vi "Control.vi"(8 "DAQ Status":T1, 11 "UI Refs":T6) -> (0 "WaveGen Action":T5, 1 "WaveGen Params":T4, 4 "DAQ Params":T2, 6 "DAQ Action":T3)   [LabVIEW 2020, in "DAQ AO SFP.lvlib"]
uses:
  DAQ AO SFP.lvlib
  UI Refs.ctl
  <extravilib>/ChannelInstances/Flex-t'WaveGen.lvlib-Gen Action.ctl'/))Channel.ctl
  WaveGen/Gen Action.ctl
  <extravilib>/ChannelInstances/Flex-t'WaveGen.lvlib-Gen Params.ctl'/))Channel.ctl
  WaveGen/Gen Params.ctl
  WaveGen/Timing Params.ctl
  WaveGen/Signal Params.ctl
  WaveGen/Shape.ctl
  <extravilib>/ChannelInstances/Flex-t'DAQmx AO.lvlib-Action.ctl'/))Channel.ctl
  DAQmx AO/Action.ctl
  <extravilib>/ChannelInstances/Flex-t'DAQmx AO.lvlib-Params.ctl'/))Channel.ctl
  DAQmx AO/Params.ctl
  <extravilib>/ChannelInstances/Flex-t'DAQmx AO.lvlib-Status.ctl'/))Channel.ctl
  DAQmx AO/Status.ctl
  <extravilib>/ChannelInstances/Flex-t'DAQmx AO.lvlib-Status.ctl'/Event Data.ctl
  <extravilib>/ChannelInstances/Flex-t'DAQmx AO.lvlib-Status.ctl'.lvlib
  DAQmx AO/DAQmx AO.lvlib
  WaveGen/WaveGen.lvlib
  <extravilib>/ChannelInstances/Flex-t'DAQmx AO.lvlib-Params.ctl'.lvlib
  <extravilib>/ChannelInstances/Flex-t'WaveGen.lvlib-Gen Params.ctl'.lvlib
  <extravilib>/ChannelInstances/Flex-t'DAQmx AO.lvlib-Action.ctl'.lvlib
  <extravilib>/ChannelInstances/Flex-t'WaveGen.lvlib-Gen Action.ctl'.lvlib
panel:
  out "Valid":bool
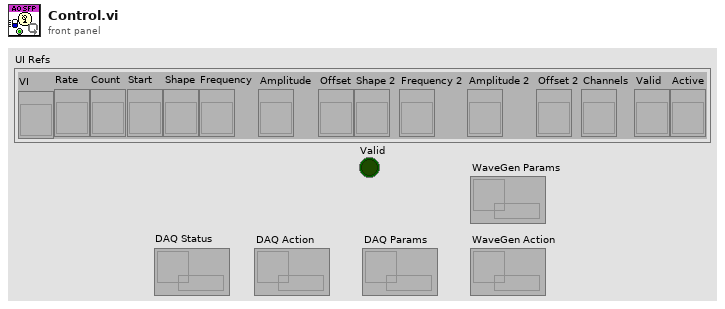
[diagram p1: front panel]
types:
  T1 = typedef "Flex-t'DAQmx AO.lvlib-Status.ctl'.lvlib/))Channel.ctl" = refnum<queue>
  T2 = typedef "Flex-t'DAQmx AO.lvlib-Params.ctl'.lvlib/))Channel.ctl" = refnum<queue>
  T3 = typedef "Flex-t'DAQmx AO.lvlib-Action.ctl'.lvlib/))Channel.ctl" = refnum<queue>
  T4 = typedef "Flex-t'WaveGen.lvlib-Gen Params.ctl'.lvlib/))Channel.ctl" = refnum<queue>
  T5 = typedef "Flex-t'WaveGen.lvlib-Gen Action.ctl'.lvlib/))Channel.ctl" = refnum<queue>
  T6 = typedef "DAQ AO SFP.lvlib/UI Refs.ctl" = cluster{"VI":refnum<vi>, "Rate":refnum<vi>, "Count":refnum<vi>, "Start":refnum<vi>, "Shape":refnum<vi>, "Frequency":refnum<vi>, "Amplitude":refnum<vi>, "Offset":refnum<vi>, "Shape 2":refnum<vi>, "Frequency 2":refnum<vi>, "Amplitude 2":refnum<vi>, "Offset 2":refnum<vi>, "Channels":refnum<vi>, "Valid":refnum<vi>, "Active":refnum<vi>}
  T7 = cluster{"DAQ Status":refnum<event-registration>, "Event Registration Refnum":refnum<event-registration>}
  T8 = typedef "WaveGen.lvlib/Gen Action.ctl" = enum16{"Run Once", "Generate", "Close", "Stop"}
  T9 = typedef "DAQmx AO.lvlib/Action.ctl" = enum16{"Verify", "Start", "Stop", "Close", "Error"}
  T10 = typedef "WaveGen.lvlib/Gen Params.ctl" = cluster{"Timing Params":T11, "Signal Params":T12[]}
  T11 = typedef "WaveGen.lvlib/Timing Params.ctl" = cluster{"Sample Rate":dbl, "Sample Count":dbl}
  T12 = typedef "WaveGen.lvlib/Signal Params.ctl" = cluster{"Shape":T13, "Frequency":dbl, "Amplitude":dbl, "Offset":dbl, "Phase":dbl}
  T13 = typedef "WaveGen.lvlib/Shape.ctl" = enum16{"Sine", "Square", "Triangle", "Saw"}
  T14 = typedef "DAQmx AO.lvlib/Params.ctl" = cluster{"Channels":tag, "Sample Rate":dbl, "Sample Count":i32}
  T15 = typedef "DAQmx AO.lvlib/Status.ctl" = cluster{"Valid":bool, "Active":bool}
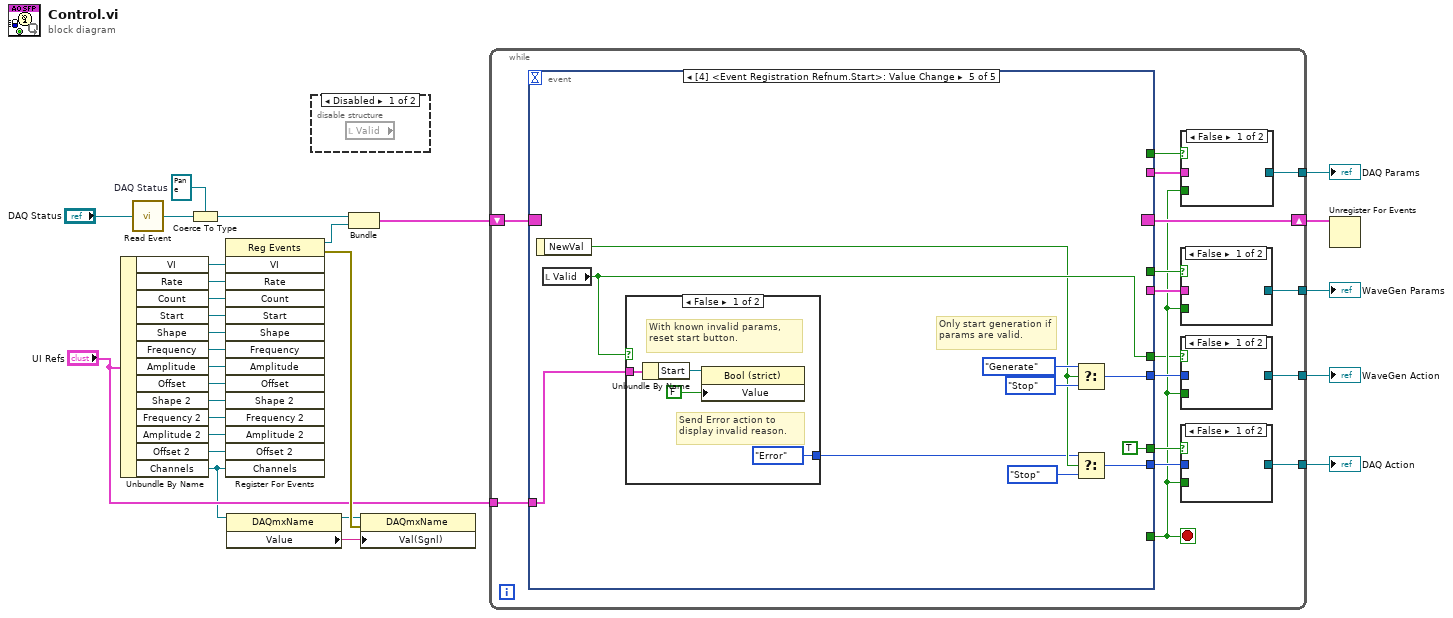
[diagram p0: block diagram]
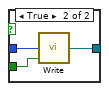
[diagram p3: hidden frame]
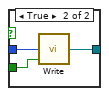
[diagram p4: hidden frame]
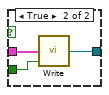
[diagram p5: hidden frame]
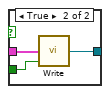
[diagram p6: hidden frame]
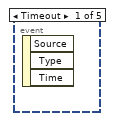
[diagram p7: hidden frame]
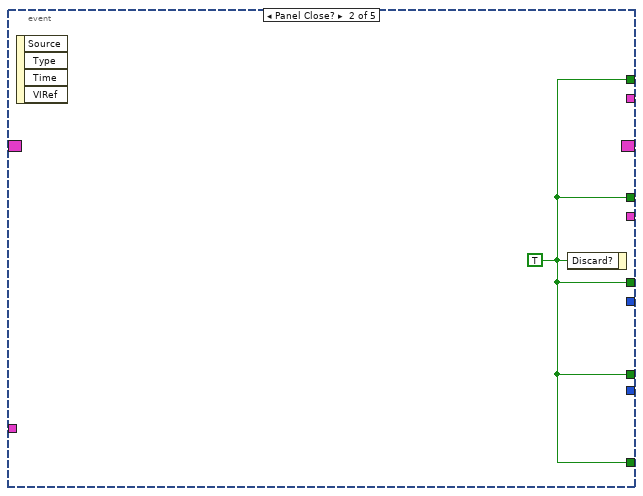
[diagram p8: hidden frame]
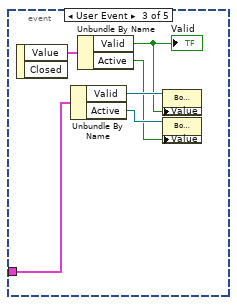
[diagram p9: hidden frame]
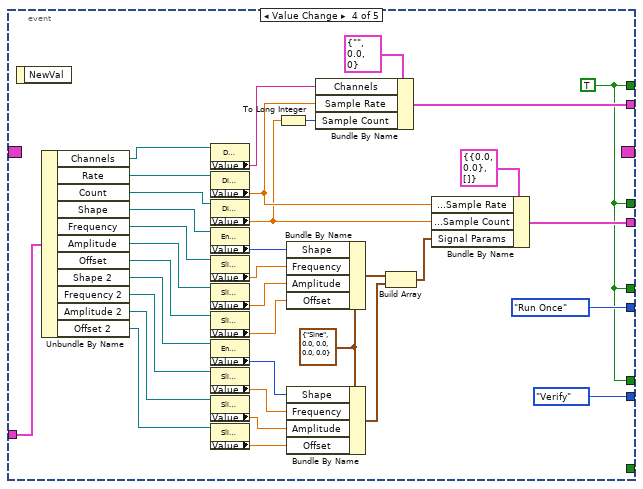
[diagram p10: hidden frame]
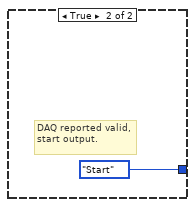
[diagram p11: hidden frame]
diagram:
  w12 = refnum<event-registration> refnum  # DAQ Status
  n1 = Unbundle By Name("UI Refs") -> ("VI"=w27:refnum<vi>, "Rate"=w26:refnum<vi>, "Count"=w25:refnum<vi>, "Start"=w24:refnum<vi>, "Shape"=w23:refnum<vi>, "Frequency"=w22:refnum<vi>, "Amplitude"=w21:refnum<vi>, "Offset"=w20:refnum<vi>, "Shape 2"=w19:refnum<vi>, "Frequency 2"=w18:refnum<vi>, "Amplitude 2"=w17:refnum<vi>, "Offset 2"=w16:refnum<vi>, "Channels"=w3:refnum<vi>)
  n2 = call <extravilib>:"Read Event.vi"("FlexChannel"="DAQ Status") -> ("Event Reg"=w13:refnum<event-registration>)  [unwired: 8 in]
  n3 = Coerce To Type(0:w13, 1:w12) -> (2:w11:refnum<event-registration>)
  n4 = register-events(w27, w26, w25, w24, w23, w22, w21, w20, w19, w18, w17, w16, w3) -> (reference out=w10:refnum<event-registration>, error out=w28:errorcluster)  [unwired: 2 in]
  n5 = property class="DAQmxName"(reference=w3) -> (reference out=w2:refnum<vi>, "Value"=w1:string)  [unwired: 1 in, 1 out]
  n6 = disable-structure shown="Disabled" {
    frame Disabled {
      n7 = local read "Valid"() -> ()  [unwired: 1 out]
    }
    frame Enabled {
    }
  }
  n8 = Bundle("DAQ Status"=w11, "Event Registration Refnum"=w10) -> (w9:T7)  [unwired: 1 in]
  n9 = property class="DAQmxName"(reference=w2, error in=w28, "Val(Sgnl)"=w1) -> ()  [unwired: 2 out]
  n10 = while {
    shift-right: [w43] -> w15
    shift-left: w9 -> [w44]
    tunnel: "UI Refs" -> [w42]
    tunnel: [w41] -> w7
    tunnel: [w38] -> w6
    tunnel: [w35] -> w5
    tunnel: [w32] -> w4
    stop <- w30 stop-if-true
    n11 = event shown="[4] <Event Registration Refnum.Start>: Value Change" {
      selector: w44 -> [_ _ _ _ _]
      dyn-events: [_ _ _ _ _] -> w43
      timeout: _ -> [_ _ _ _ _]
      tunnel: w42 -> [_ _ w63 w98 w103]
      tunnel: [_ _ _ w81 _] -> w40
      tunnel: [_ w57 _ w64 _] -> w39
      tunnel: [_ w57 _ _ _] -> w30
      tunnel: [_ w57 _ w64 _] -> w37
      tunnel: [_ _ _ w67 _] -> w36
      tunnel: [_ _ _ Action."Verify" ("element") w105] -> w34
      tunnel: [_ w57 _ w64 TRUE ("Discard?")] -> w33
      tunnel: [_ _ _ Gen_Action."Run Once" ("element") w108] -> w31
      tunnel: [_ w57 _ w64 w102] -> w29
      event Timeout {
        n12 = event-data() -> ()  [unwired: 1 in, 3 out]
      }
      event Panel Close? {
        w57 = TRUE ("Discard?")
        n13 = event-data() -> ()  [unwired: 1 in, 4 out]
        n14 = event-data("Discard?"=w57) -> ()  [unwired: 1 in, 1 out]
      }
      event User Event {
        n15 = event-data() -> ("Value"=w60:T15)  [unwired: 1 in, 1 out]
        n16 = Unbundle By Name(w63) -> ("Valid"=w61:refnum<vi>, "Active"=w62:refnum<vi>)
        n17 = Unbundle By Name(w60) -> ("Valid"=w58:bool, "Active"=w59:bool)
        "Valid" <- w58
        n18 = property class="Bool (strict)"(reference=w61, "Value"=w58) -> ()  [unwired: 1 in, 2 out]
        n19 = property class="Bool (strict)"(reference=w62, "Value"=w59) -> ()  [unwired: 1 in, 2 out]
      }
      event Value Change {
        w76 = T12 {"Shape"=enum."Sine", "Frequency"=0.0, "Amplitude"=0.0, "Offset"=0.0, "Phase"=0.0} ("Signal Params")
        w64 = TRUE
        n20 = event-data() -> ()  [unwired: 1 in, 1 out]
        n21 = Unbundle By Name(w98) -> ("Channels"=w87:refnum<vi>, "Rate"=w97:refnum<vi>, "Count"=w96:refnum<vi>, "Shape"=w95:refnum<vi>, "Frequency"=w94:refnum<vi>, "Amplitude"=w93:refnum<vi>, "Offset"=w92:refnum<vi>, "Shape 2"=w91:refnum<vi>, "Frequency 2"=w90:refnum<vi>, "Amplitude 2"=w89:refnum<vi>, "Offset 2"=w88:refnum<vi>)
        n22 = property class="DAQmxName"(reference=w87) -> ("Value"=w85:string)  [unwired: 1 in, 2 out]
        n23 = property class="DigNum (strict)"(reference=w97) -> ("Value"=w83:dbl)  [unwired: 1 in, 2 out]
        n24 = property class="DigNum (strict)"(reference=w96) -> ("Value"=w82:dbl)  [unwired: 1 in, 2 out]
        n25 = property class="Enum (strict)"(reference=w95) -> ("Value"=w75:T13)  [unwired: 1 in, 2 out]
        n26 = property class="Slide (strict)"(reference=w94) -> ("Value"=w74:dbl)  [unwired: 1 in, 2 out]
        n27 = property class="Slide (strict)"(reference=w93) -> ("Value"=w73:dbl)  [unwired: 1 in, 2 out]
        n28 = property class="Slide (strict)"(reference=w92) -> ("Value"=w72:dbl)  [unwired: 1 in, 2 out]
        n29 = property class="Enum (strict)"(reference=w91) -> ("Value"=w77:T13)  [unwired: 1 in, 2 out]
        n30 = property class="Slide (strict)"(reference=w90) -> ("Value"=w78:dbl)  [unwired: 1 in, 2 out]
        n31 = property class="Slide (strict)"(reference=w89) -> ("Value"=w79:dbl)  [unwired: 1 in, 2 out]
        n32 = property class="Slide (strict)"(reference=w88) -> ("Value"=w80:dbl)  [unwired: 1 in, 2 out]
        n33 = To Long Integer(number=w82) -> (32bit integer=w84:i32)
        n34 = Bundle By Name(cluster=w76, "Shape"=w75, "Frequency"=w74, "Amplitude"=w73, "Offset"=w72) -> (w71:T12)
        n35 = Bundle By Name(cluster=w76, "Shape"=w77, "Frequency"=w78, "Amplitude"=w79, "Offset"=w80) -> (w70:T12)
        n36 = Bundle By Name(cluster=T14 {"Channels"="", "Sample Rate"=0.0, "Sample Count"=0} ("Params"), "Channels"=w85, "Sample Rate"=w83, "Sample Count"=w84) -> (w81:T14)
        n37 = Build Array(w71, w70) -> (w69:T12[])
        n38 = Bundle By Name(cluster=T10 {"Timing Params"={"Sample Rate"=0.0, "Sample Count"=0.0}, "Signal Params"=[]} ("Gen Params"), "Timing Params.Sample Rate"=w83, "Timing Params.Sample Count"=w82, "Signal Params"=w69) -> (w67:T10)
      }
      event Value Change {
        # "Only start generation if params are valid."
        n39 = event-data() -> ("NewVal"=w101:bool)  [unwired: 1 in]
        n40 = local read "Valid"() -> (w102:bool)
        n41 = case shown="False" w102 {
          tunnel: w103 -> [w112 _]
          tunnel: [Action."Error" ("element") Action."Start" ("element")] -> w99
          frame False {
            # "Send Error action to display invalid reason."
            # "With known invalid params, reset start button."
            n42 = Unbundle By Name(w112) -> ("Start"=w111:refnum<vi>)
            n43 = property class="Bool (strict)"(reference=w111, "Value"=FALSE) -> ()  [unwired: 1 in, 2 out]
          }
          frame True {
            # "DAQ reported valid, start output."
          }
        }
        n44 = Select(t=Gen_Action."Generate" ("element"), s=w101, f=Gen_Action."Stop" ("element")) -> (s? t:f=w108:T8)
        n45 = Select(t=w99, s=w101, f=Action."Stop" ("element")) -> (s? t:f=w105:T9)
      }
    }
    n46 = case shown="False" w39 {
      tunnel: [_ w56] -> w41
      tunnel: w40 -> [_ w55]
      tunnel: w30 -> [_ w54]
      frame False {
      }
      frame True {
        n47 = call <extravilib>:"Write.vi"("element"=w55, "Close? (F)"=w54) -> ("channel"=w56:T2)  [unwired: 5 in, 2 out]
      }
    }
    n48 = case shown="False" w37 {
      tunnel: [_ w53] -> w38
      tunnel: w36 -> [_ w52]
      tunnel: w30 -> [_ w51]
      frame False {
      }
      frame True {
        n49 = call <extravilib>:"Write.vi"("element"=w52, "Close? (F)"=w51) -> ("channel"=w53:T4)  [unwired: 5 in, 2 out]
      }
    }
    n50 = case shown="False" w29 {
      tunnel: [_ w47] -> w32
      tunnel: w31 -> [_ w46]
      tunnel: w30 -> [_ w45]
      frame False {
      }
      frame True {
        n51 = call <extravilib>:"Write.vi"("element"=w46, "Close? (F)"=w45) -> ("channel"=w47:T5)  [unwired: 5 in, 2 out]
      }
    }
    n52 = case shown="False" w33 {
      tunnel: [_ w50] -> w35
      tunnel: w34 -> [_ w49]
      tunnel: w30 -> [_ w48]
      frame False {
      }
      frame True {
        n53 = call <extravilib>:"Write.vi"("element"=w49, "Close? (F)"=w48) -> ("channel"=w50:T3)  [unwired: 5 in, 2 out]
      }
    }
  }
  "WaveGen Action" <- w4
  "WaveGen Params" <- w6
  "DAQ Action" <- w5
  "DAQ Params" <- w7
  n54 = Unregister For Events(event registration refnum=w15) -> ()  [unwired: 1 in, 1 out]
